vi "BASIC_SUBVI_LoadDataWithColumnName.vi"(4 "error in (no error)":errorcluster, 7 "path in":path) -> (0 "error out":errorcluster, 1 "2D data":dbl[][](array[numeric]) format="%0.2f", 2 "column names":string[](array[string]), 3 "path out":path)   [LabVIEW 2020, in "BasicVIs.lvlib"]
uses:
  BasicVIs.lvlib
  <vilib>/Utility/error.llb/whitespace.ctl
  <vilib>/Utility/file.llb/Read From Spreadsheet File (DBL).vi
panel:
  out "#column name":i32
  out "#data column":i32
  out "error?":string
  out "chars":string[](array[string])
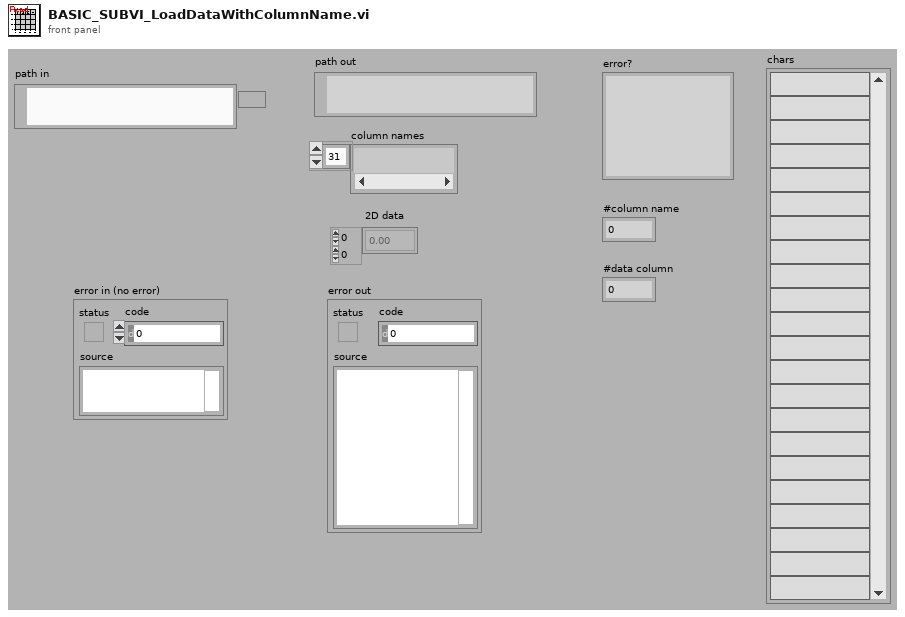
[diagram p1: front panel]
types:
  T1 = typedef "whitespace.ctl" = u16
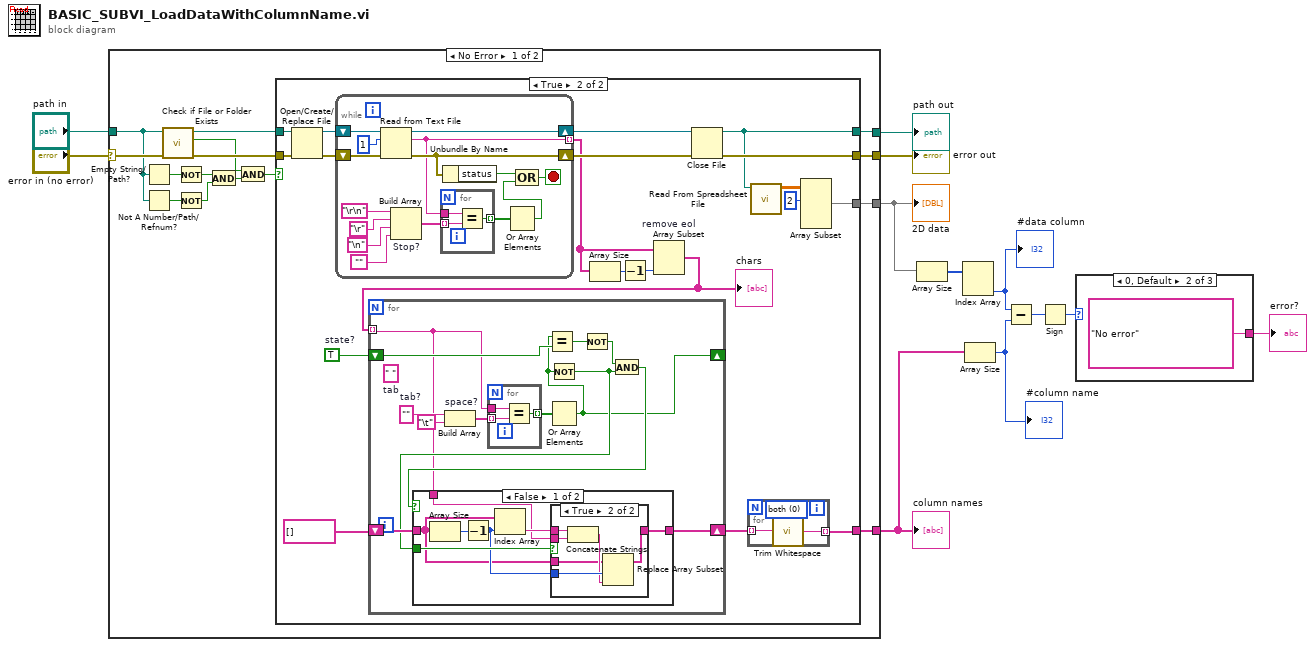
[diagram p0: block diagram]
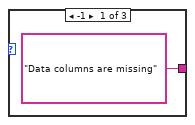
[diagram p2: hidden frame]
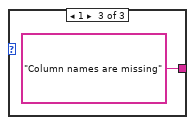
[diagram p3: hidden frame]
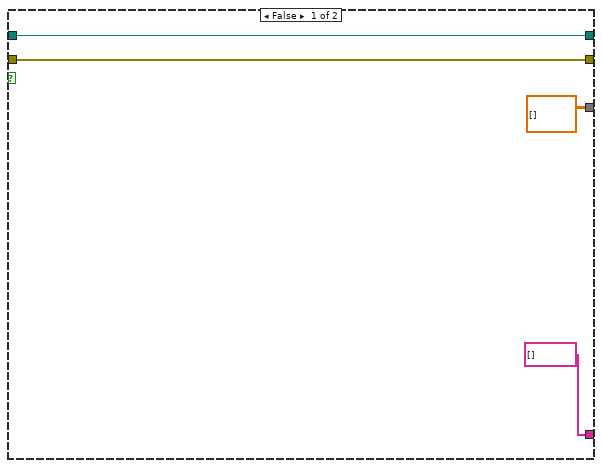
[diagram p4: hidden frame]
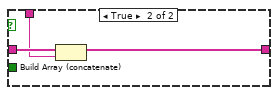
[diagram p6: hidden frame]
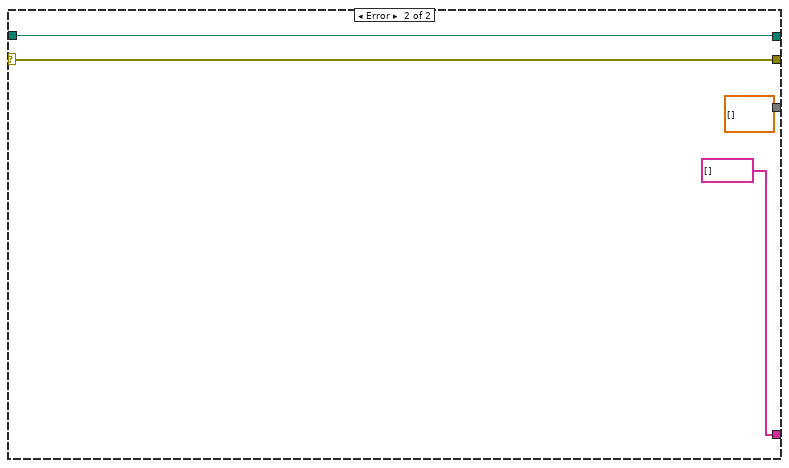
[diagram p7: hidden frame]
diagram:
  n1 = case shown="No Error" "error in (no error)" {
    selector: "error in (no error)" -> [w25 w108]
    tunnel: "path in" -> [w19 w107]
    tunnel: [w16 w107] -> w11
    tunnel: [w15 w108] -> w10
    tunnel: [w14 dbl[][] []] -> w8
    tunnel: [w13 string[] [] ("Column name array")] -> w6
    frame No Error {
      n2 = Empty String/Path?(string/path=w19) -> (empty?=w23:bool)
      n3 = Not A Number/Path/Refnum?(number/path/refnum=w19) -> (NaN/Path/Refnum?=w24:bool)
      n4 = call <vilib>:"Check if File or Folder Exists.vi"("error in (no error)"=w25, "path"=w19) -> ("error out"=w26:errorcluster, "file or folder exists?"=w18:bool, "dup path"=w27:path)  [unwired: 7 in]
      n5 = Not(x=w23) -> (.not. x?=w22:bool)
      n6 = Not(x=w24) -> (.not. x?=w21:bool)
      n7 = And(x=w22, y=w21) -> (x .and. y?=w20:bool)
      n8 = And(x=w18, y=w20) -> (x .and. y?=w17:bool)
      n9 = case shown="True" w17 {
        tunnel: w27 -> [w30 w46]
        tunnel: w26 -> [w31 w45]
        tunnel: [w30 w40] -> w16
        tunnel: [w31 w44] -> w15
        tunnel: [dbl[][] [] w41] -> w14
        tunnel: [string[] [] w32] -> w13
        frame False {
        }
        frame True {
          w38 = TRUE  # state?
          n10 = Open/Create/Replace File(file path (use dialog)=w46, error in=w45) -> (refnum out=w50:refnum<file>, error out=w49:errorcluster)  [unwired: 4 in, 1 out]
          n11 = while {
            shift-right: [w99] -> w48
            shift-left: w50 -> [w101]
            shift-right: [w96] -> w47
            shift-left: w49 -> [w100]
            tunnel: [w89] -> w34 mode=indexing
            stop <- w97 stop-if-true
            n12 = Read from Text File(file (use dialog)=w101, count=1, error in=w100) -> (refnum out=w99:refnum<file>, text=w89:string, error out=w96:errorcluster)  [unwired: 1 in, 1 out]
            n13 = Build Array "Stop?"("\r\n", "\r", "\n", "") -> (w90:string[])
            n14 = for {
              tunnel: w90 -> [w103] mode=indexing
              tunnel: w89 -> [w104]
              tunnel: [w102] -> w88 mode=indexing
              n15 = Equal?(x=w104, y=w103) -> (x = y?=w102:bool)
            }
            n16 = Unbundle By Name(w96) -> ("status"=w95:bool)
            n17 = Or Array Elements(Boolean array=w88) -> (logical OR=w87:bool)
            n18 = Compound Arithmetic op=OR(w95, w87) -> (w97:bool)
          }
          n19 = Array Size(array=w34) -> (size(s)=w37:i32)
          n20 = Decrement(x=w37) -> (x-1=w36:i32)
          n21 = Array Subset "remove eol"(array=w34, length=w36) -> (w35:string[])  [unwired: 1 in]
          "chars" <- w35
          n22 = for {
            tunnel: w35 -> [w56] mode=indexing
            shift-right: [w62] -> w33
            shift-left: string[] [] -> [w63]
            shift-right: [w54] -> _
            shift-left: w38 -> [w66]
            w58 = ""  # tab?
            (unwired) " "  # tab
            n23 = Build Array "space?"(w58, "\t") -> (w59:string[])
            n24 = for {
              tunnel: w59 -> [w68] mode=indexing
              tunnel: w56 -> [w69]
              tunnel: [w67] -> w55 mode=indexing
              n25 = Equal?(x=w69, y=w68) -> (x = y?=w67:bool)
            }
            n26 = Or Array Elements(Boolean array=w55) -> (logical OR=w54:bool)
            n27 = Equal?(x=w54, y=w66) -> (x = y?=w65:bool)
            n28 = Not(x=w54) -> (.not. x?=w60:bool)
            n29 = Not(x=w65) -> (.not. x?=w64:bool)
            n30 = And(x=w64, y=w60) -> (x .and. y?=w61:bool)
            n31 = case shown="False" w61 {
              tunnel: w63 -> [w71 w86]
              tunnel: [w70 w85] -> w62
              tunnel: w56 -> [w72 w84]
              tunnel: w60 -> [w76 _]
              frame False {
                n32 = Array Size(array=w71) -> (size(s)=w75:i32)
                n33 = Decrement(x=w75) -> (x-1=w74:i32)
                n34 = Index Array(array=w71, index=w74) -> (element=w73:string)
                n35 = case shown="True" w76 {
                  tunnel: w74 -> [_ w83]
                  tunnel: w73 -> [_ w82]
                  tunnel: w72 -> [_ w81]
                  tunnel: w71 -> [w77 w79]
                  tunnel: [w77 w78] -> w70
                  frame False {
                  }
                  frame True {
                    n36 = Concatenate Strings(w82, w81) -> (w80:string)
                    n37 = Replace Array Subset(array=w79, new element=w80, index=w83) -> (w78:string[])
                  }
                }
              }
              frame True {
                n38 = Build Array (concatenate)(w86, w84) -> (w85:string[])
              }
            }
          }
          n39 = Close File(refnum=w48, error in=w47) -> (path=w40:path, error out=w44:errorcluster)
          n40 = for {
            tunnel: w33 -> [w53] mode=indexing
            tunnel: [w52] -> w32 mode=indexing
            w51 = T1 0 items=["both", "start of string", "end of string"] ("location (both)")
            n41 = call <vilib>:"Trim Whitespace.vi"("string"=w53, "location (both)"=w51) -> ("trimmed string"=w52:string)
          }
          n42 = call-poly <vilib>:"Read From Spreadsheet File.vi"("file path (dialog if empty)"=w40) -> ("all rows"=w42:dbl[][])  [unwired: 6 in, 4 out]
          n43 = Array Subset(array=w42, index (row)=2 ("index")) -> (w41:dbl[][])  [unwired: 3 in]
        }
      }
    }
    frame Error {
    }
  }
  "2D data" <- w8
  "path out" <- w11
  "column names" <- w6
  "error out" <- w10
  n44 = Array Size(array=w8) -> (size(s)=w7:i32[])
  n45 = Index Array(array=w7) -> (element #2=w5:i32)  [unwired: 2 in, 1 out]
  "#data column" <- w5
  n46 = Array Size(array=w6) -> (size(s)=w1:i32)
  "#column name" <- w1
  n47 = Subtract(x=w5, y=w1) -> (x-y=w4:i32)
  n48 = Sign(1:w4) -> (0:w3:i32)
  n49 = case shown="0, Default" w3 {
    tunnel: ["Data columns are missing" "No error" "Column names are missing"] -> w2
    frame -1 {
    }
    frame 0, Default {
    }
    frame 1 {
    }
  }
  "error?" <- w2
